vi "StackMeanCI_subvi.vi"(11 "Stack":dbl[][](array[numeric])) -> (3 "Three Lines":dbl[][](array[numeric]))   [LabVIEW 2019]
uses:
  <vilib>/Analysis/baseanly.llb/Mean (DBL).vi
  <vilib>/Analysis/NI_AALBase.lvlib
  <vilib>/gmath/NI_Gmath.lvlib
panel:
  out "size(s)":i32
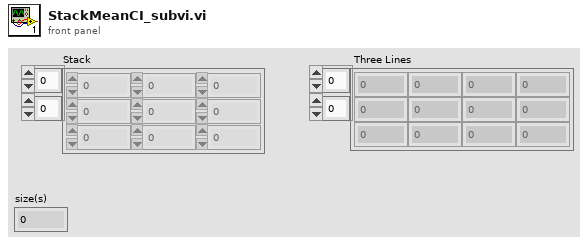
[diagram p1: front panel]
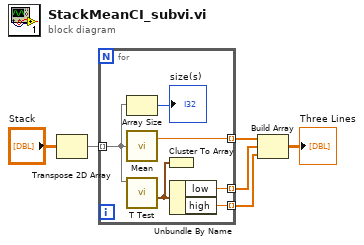
[diagram p0: block diagram]
diagram:
  n1 = Transpose 2D Array(2D array="Stack") -> (transposed array=w2:dbl[][])
  n2 = for {
    tunnel: w2 -> [w10] mode=indexing
    tunnel: [w12] -> w6 mode=indexing
    tunnel: [w8] -> w5 mode=indexing
    tunnel: [w7] -> w4 mode=indexing
    n3 = Array Size(array=w10) -> (size(s)=→"size(s)":i32)
    n4 = call-poly <vilib>:"Mean.vi"("X"=w10) -> ("mean"=w12:dbl)  [unwired: 1 out]
    n5 = call <vilib>:"T Test.vi"("sample set"=w10) -> ("confidence interval"=w9:cluster{"low":dbl, "high":dbl})  [unwired: 6 in, 4 out]
    n6 = Cluster To Array(cluster=w9) -> ()  [unwired: 1 out]
    n7 = Unbundle By Name(w9) -> ("low"=w8:dbl, "high"=w7:dbl)
  }
  n8 = Build Array(w6, w5, w4) -> (→"Three Lines":dbl[][])
